vi "ExecuteSkill.vi"() -> ()   [LabVIEW 2023, in "GoToOneShotPosition.lvclass"]
uses:
  GoToOneShotPosition.lvclass
  Game_class/Game.lvclass
  Field_class/Field.lvclass
  Utilities_class/Utilities.lvclass
  NewSTP/NewSkills/GoToTargetPositionSkill_class/GoToTargetPositionSkill.lvclass
  <vilib>/Analysis/NI_AALBase.lvlib
  <vilib>/Analysis/baseanly.llb/Unit Vector (DBL).vi
  Robot_class/Robot.lvclass
  Zone_class/Zone.lvclass
panel:
  in  "RobotSize":dbl
  out "Robot out":refnum<class "Robot.lvclass">
  in  "GameRef":refnum<data-value>
  in  "Robot in":refnum<class "Robot.lvclass">
  out "object out":refnum<class "GoToTargetPositionSkill.lvclass">
  in  "object in":refnum<class "GoToTargetPositionSkill.lvclass">
  out "error out":errorcluster
  in  "error in (no error)":errorcluster
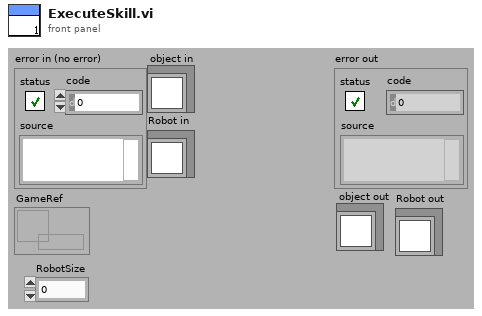
[diagram p1: front panel]
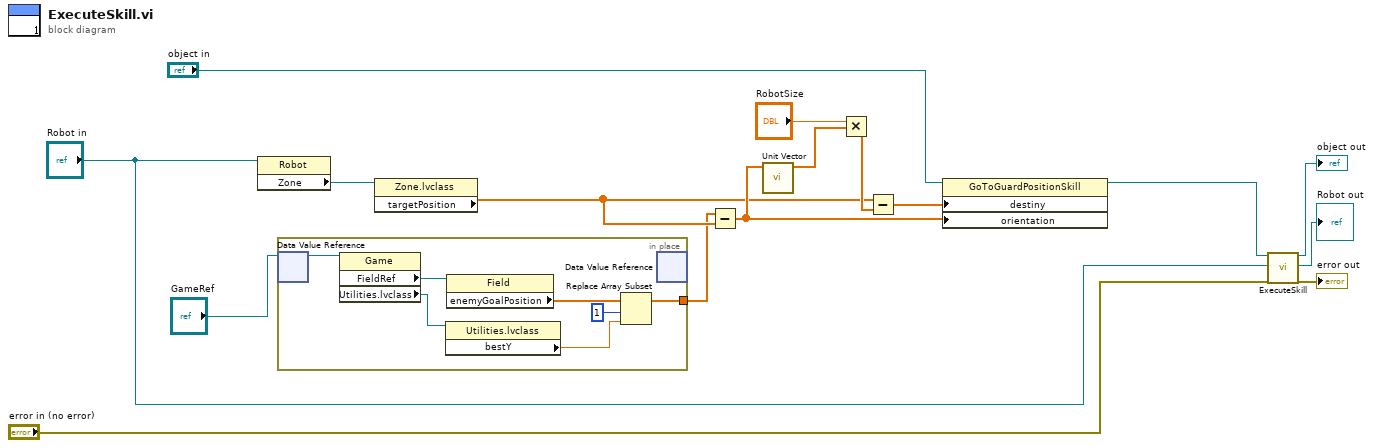
[diagram p0: block diagram]
diagram:
  n1 = property class="Robot"(reference="Robot in") -> ("Zone"=w10:refnum<class "Zone.lvclass">)  [unwired: 1 in, 2 out]
  n2 = in-place {
    in-place-border: [w19] -> w1
    n3 = in-place-dvr #1("GameRef") -> (w23:refnum<class "Game.lvclass">)  [unwired: 1 out]
    n4 = property class="Game"(reference=w23) -> ("FieldRef"=w22:refnum<class "Field.lvclass">, "Utilities.lvclass"=w21:refnum<class "Utilities.lvclass">)  [unwired: 1 in, 2 out]
    n5 = property class="Utilities.lvclass"(reference=w21) -> ("bestY"=w18:dbl)  [unwired: 1 in, 2 out]
    n6 = property class="Field"(reference=w22) -> ("enemyGoalPosition"=w20:dbl[])  [unwired: 1 in, 2 out]
    n7 = Replace Array Subset(array=w20, new element=w18, index=1) -> (w19:dbl[])
    n8 = in-place-dvr #1() -> ()  [unwired: 1 in, 2 out]
  }
  n9 = property class="Zone.lvclass"(reference=w10) -> ("targetPosition"=w2:dbl[])  [unwired: 1 in, 2 out]
  n10 = Subtract(x=w1, y=w2) -> (x-y=w7:dbl[])
  n11 = call-poly <vilib>:"Unit Vector.vi"("Input Vector"=w7) -> ("Unit Vector"=w6:dbl[])  [unwired: 8 in, 2 out]
  n12 = Multiply(x="RobotSize", y=w6) -> (x*y=w4:dbl[])
  n13 = Subtract(x=w2, y=w4) -> (x-y=w3:dbl[])
  n14 = property class="GoToGuardPositionSkill"(reference="object in", "destiny"=w3, "orientation"=w7) -> (reference out=w9:refnum<class "GoToTargetPositionSkill.lvclass">)  [unwired: 1 in, 1 out]
  n15 = call-parent "ExecuteSkill.vi"("object in"=w9, "Robot in"="Robot in", "error in (no error)"="error in (no error)") -> ("object out"=→"object out":refnum<class "GoToTargetPositionSkill.lvclass">, "Robot out"=→"Robot out":refnum<class "Robot.lvclass">, "error out"=→"error out":errorcluster)  [unwired: 14 in]
